vi "SubVI_Add.vi"(9 "Kullanıcı Bilgileri":T3 {"Boy" min=1.0 max=2.5 step=0.01; "Yaş" min=10.0 max=100.0}, 10 "UID":u64, 11 "Kullanıcı Listesi in":T1) -> (3 "Kullanıcı Listesi out":T1)   [LabVIEW 2024]
uses:
  Control 2_1.ctl
  Control 3.ctl
  Documents/LabView Projects/Control 1.ctl
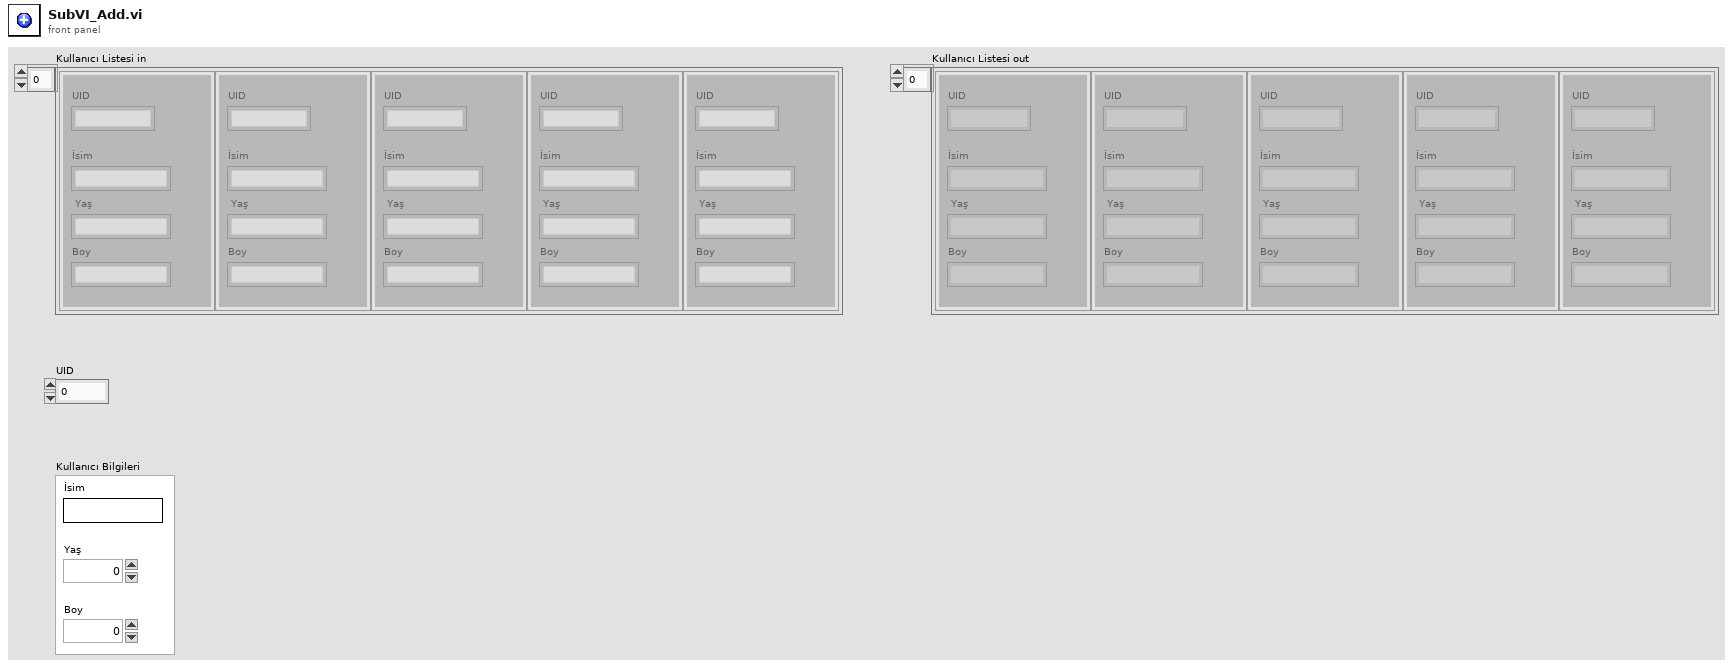
[diagram p1: front panel]
types:
  T1 = typedef "Control 3.ctl" = T2[]
  T2 = typedef "Control 1.ctl" = cluster{"UID":string, "İsim":string, " Yaş":string, "Boy":string}
  T3 = typedef "Control 2_1.ctl" = cluster{"İsim":string, "Yaş":dbl, "Boy":dbl}
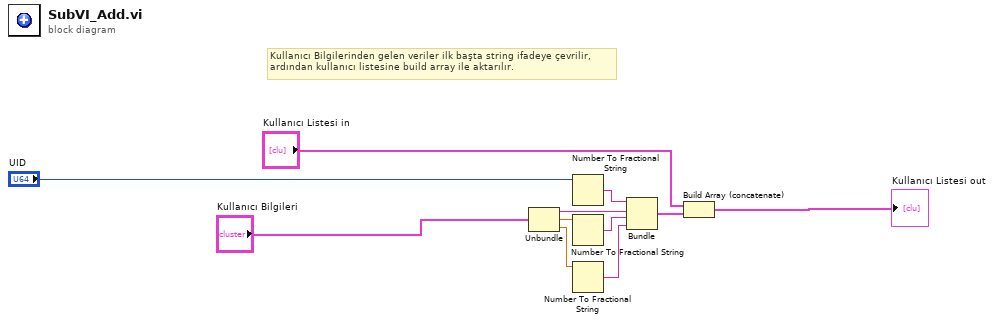
[diagram p0: block diagram]
diagram:
  # "Kullanıcı Bilgilerinden gelen veriler ilk başta string ifadeye çevrilir, \nardından kullanıcı listesine build array ile aktarılır."
  n1 = Unbundle("Kullanıcı Bilgileri") -> ("İsim"=w1:string, "Yaş"=w8:dbl, "Boy"=w10:dbl)
  n2 = Number To Fractional String(number="UID") -> (F-format string=w7:string)  [unwired: 3 in]
  n3 = Number To Fractional String(number=w8) -> (F-format string=w9:string)  [unwired: 3 in]
  n4 = Number To Fractional String(number=w10) -> (F-format string=w11:string)  [unwired: 3 in]
  n5 = Bundle(w7, "İsim"=w1, w9, w11) -> (w2:cluster{string, "İsim":string, string, string})  [unwired: 1 in]
  n6 = Build Array (concatenate)("Kullanıcı Listesi in", w2) -> (→"Kullanıcı Listesi out":T1)
